vi "Path To Grid.vi"(4 "current y":i32, 6 "current x":i32, 8 "error in (no error)":errorcluster, 10 "path references":refnum<data-value>[](array[refnum]), 11 "map reference in":refnum<data-value>) -> (0 "error out":errorcluster, 1 "path on obstacles":dbl[][](graph), 3 "map reference out":refnum<data-value>, 5 "y coordinates":i32[](array[numeric]), 7 "x coordinates":i32[](array[numeric]))   [LabVIEW 2012]
uses:
  <vilib>/robotics/Navigation/shared/MapNode/AbstractAstarNode/NI_Robotics_AbstractAstarNode.lvclass
  <vilib>/robotics/Navigation/shared/WorldMap/OccupancyGridWorldMap/NI_Robotics_OccupancyGridWorldMap.lvclass
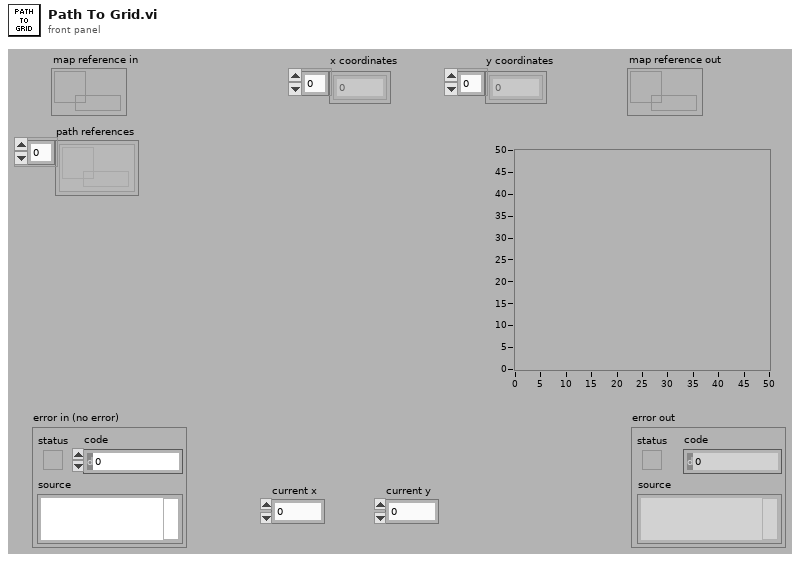
[diagram p1: front panel]
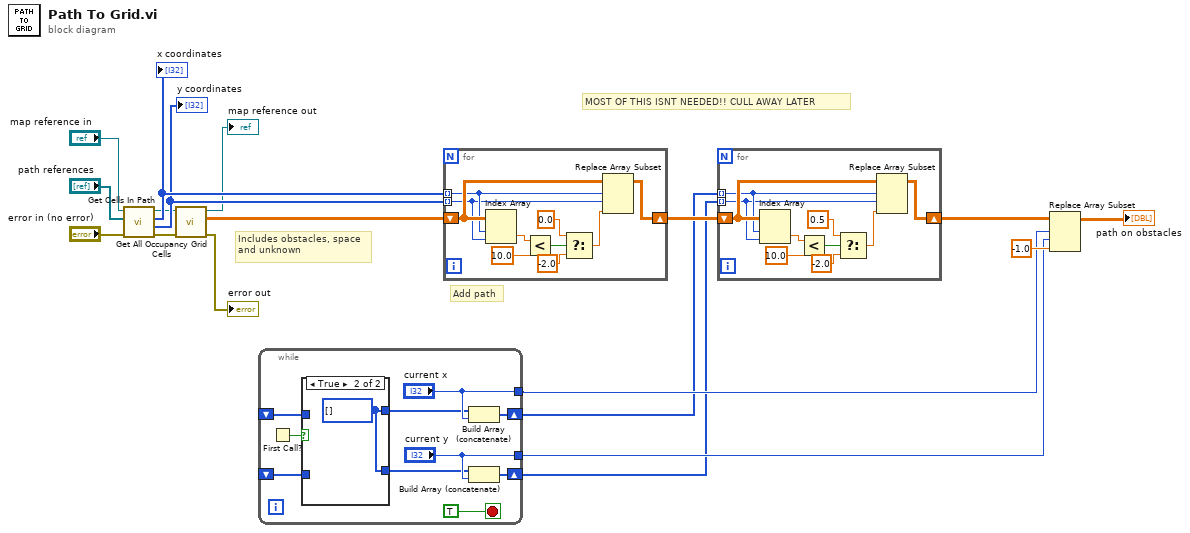
[diagram p0: block diagram]
diagram:
  # "MOST OF THIS ISNT NEEDED!! CULL AWAY LATER"
  # "Add path"
  # "Includes obstacles, space\nand unknown"
  n1 = call <vilib>:"Get Cells In Path.vi"("error in (no error)"="error in (no error)", "path references"="path references", "map reference in"="map reference in") -> ("error out"=w11:errorcluster, "y coordinates"=w17:i32[], "x coordinates"=w18:i32[], "map reference out"=w13:refnum<data-value>)  [unwired: 5 in]
  "x coordinates" <- w18
  "y coordinates" <- w17
  n2 = call <vilib>:"Get All Occupancy Grid Cells.vi"("error in (no error)"=w11, "map reference in"=w13) -> ("error out"=→"error out":errorcluster, "occupancy grid"=w14:dbl[][], "map reference out"=→"map reference out":refnum<data-value>)  [unwired: 7 in]
  n3 = while {
    tunnel: ["current y"] -> w6
    tunnel: ["current x"] -> w5
    shift-right: [w26] -> w2
    shift-left: _ -> [w23]
    shift-right: [w24] -> w1
    shift-left: _ -> [w22]
    stop <- TRUE stop-if-true
    n4 = First Call?() -> (First Call?: T/F=w21:bool)
    n5 = case shown="True" w21 {
      tunnel: w23 -> [w30 _]
      tunnel: w22 -> [w29 _]
      tunnel: [w30 w31] -> w20
      tunnel: [w29 w31] -> w19
      frame False {
      }
      frame True {
        w31 = i32[] []
      }
    }
    n6 = Build Array (concatenate)(w20, "current x") -> (w26:i32[])
    n7 = Build Array (concatenate)(w19, "current y") -> (w24:i32[])
  }
  n8 = for {
    shift-right: [w41] -> w4
    shift-left: w14 -> [w40]
    tunnel: w18 -> [w39] mode=indexing
    tunnel: w17 -> [w38] mode=indexing
    n9 = Index Array(array=w40, index (row)=w39, index (col)=w38) -> (element=w36:dbl)
    n10 = Less?(x=w36, y=10.0) -> (x < y?=w35:bool)
    n11 = Select(t=0.0 ("new element/subarray"), s=w35, f=-2.0 ("new element/subarray")) -> (s? t:f=w33:dbl)
    n12 = Replace Array Subset(array=w40, new element=w33, index (row)=w39, index (col)=w38) -> (w41:dbl[][])
  }
  n13 = for {
    shift-right: [w51] -> w3
    shift-left: w4 -> [w50]
    tunnel: w2 -> [w49] mode=indexing
    tunnel: w1 -> [w48] mode=indexing
    n14 = Index Array(array=w50, index (row)=w49, index (col)=w48) -> (element=w46:dbl)
    n15 = Less?(x=w46, y=10.0) -> (x < y?=w45:bool)
    n16 = Select(t=0.5 ("new element/subarray"), s=w45, f=-2.0 ("new element/subarray")) -> (s? t:f=w43:dbl)
    n17 = Replace Array Subset(array=w50, new element=w43, index (row)=w49, index (col)=w48) -> (w51:dbl[][])
  }
  n18 = Replace Array Subset(array=w3, new element=-1.0 ("new element/subarray"), index (row)=w5, index (col)=w6) -> (→"path on obstacles":dbl[][])
